vi "capex if then.vi"() -> ()   [LabVIEW 2013]
panel:
  out "Subsystem to set":u16=5
  out "Condition true":bool=TRUE
  out "number outputs":dbl[](array[numeric])
  out "boolean outputs":bool[](array[boolean])=[TRUE, FALSE, FALSE, FALSE]
  out "evaluation value":dbl=1.0
  out "Single value":dbl=23.041248306433495
  in  "stop":bool
  out "SHared variables":dbl[](array[numeric])=[-55770.42973935589, -55770.42973935589, -55770.42973935589, -55770.42973935589, -55753.68398615968, -55753.68398615968, -55753.68398615968, 23.041248306433495]
  in  "Number of criteria":dbl=1.0
  in  "Cluster":T1={"subsystem to check"=7, "Module"=5, "Channel"=7, "criteria"=2, "evaluation value"=1.0, "Subsystem to set"=5, "Set value"=1.0, "Set channel"=0, "Set module"=1} {"Set module" items=["Mod1"=1, "Mod2"=2, "Mod3"=3, "Mod4"=4, "Mod5"=5]; "Set channel" items=["1", "2", "3", "4", "5", "6", "7", "8", "9", "10", "11", "12", "13", "14", "15", "16", "17", "18", "19", "20", "21", "22", "23", "24", "25", "26", "27", "28", "29", "30", "31", "32"]; "Subsystem to set" items=["GPIO"=0, "Chamber temperature"=1, "Chiller"=2, "Analog out"=3, "DC volts"=5, "AC volts"=6, "Relays"=8]; "criteria" items=["==", "!=", ">", "<", ">=", "<="]; "Channel" items=["1", "2", "3", "4", "5", "6", "7", "8", "9", "10", "11", "12", "13", "14", "15", "16", "17", "18", "19", "20", "21", "22", "23", "24", "25", "26", "27", "28", "29", "30", "31", "32"]; "Module" items=["Mod1"=1, "Mod2"=2, "Mod3"=3, "Mod4"=4, "Mod5"=5]; "subsystem to check" items=["GPIO"=0, "chamber temp"=1, "chiller PV"=2, "analog in"=4, "thermocouples"=7, "disabled"=9]}
  # "error: rings need to have full complement of devices but I want to hide some"
  # "GPIO needs more work to be implemented\nSet to \"disabled\" to temporarily disable the criteria from being checked\nIf only one device, leave module set to 1"
  # "Use 0 for off\nand 1 for on\nfor relays"
  # "Little chamber = module 1\nBig chamber = module 2"
  # "gets set to"
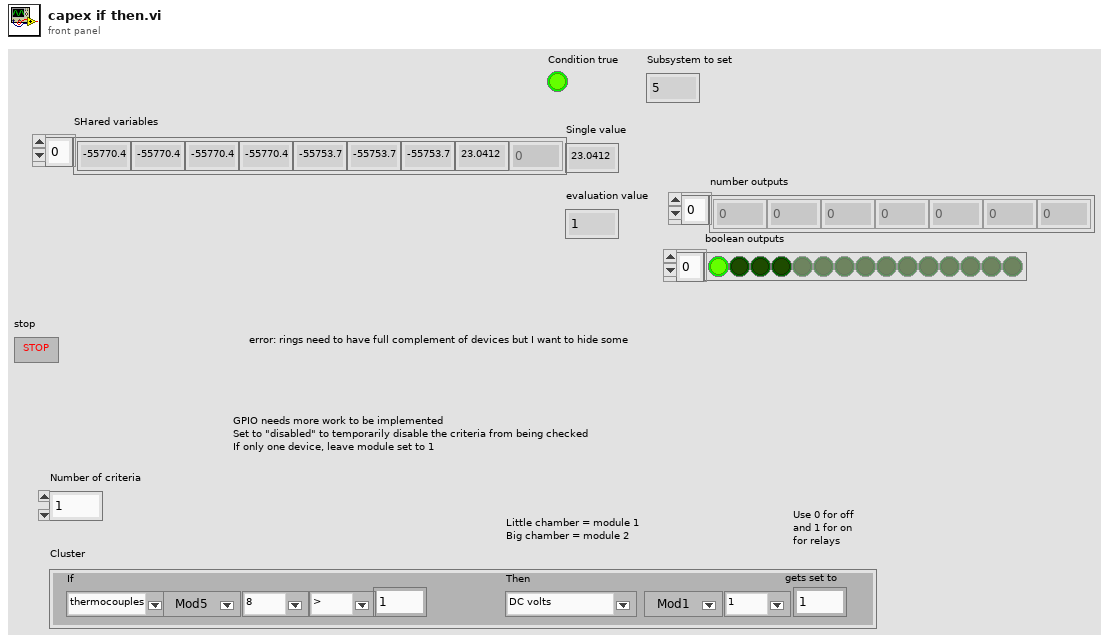
[diagram p1: front panel]
types:
  T1 = cluster{"subsystem to check":u16, "Module":u16, "Channel":u16, "criteria":u16, "evaluation value":dbl, "Subsystem to set":u16, "Set value":dbl, "Set channel":u16, "Set module":u16}
  T2 = cluster{"subsystem to check":u16, "Module":u16, "Channel":u16, "criteria":u16, "evaluation value":dbl, "Subsystem to set":u16, "Set value":dbl, "Set channel":u16, "Set module":u16}[]
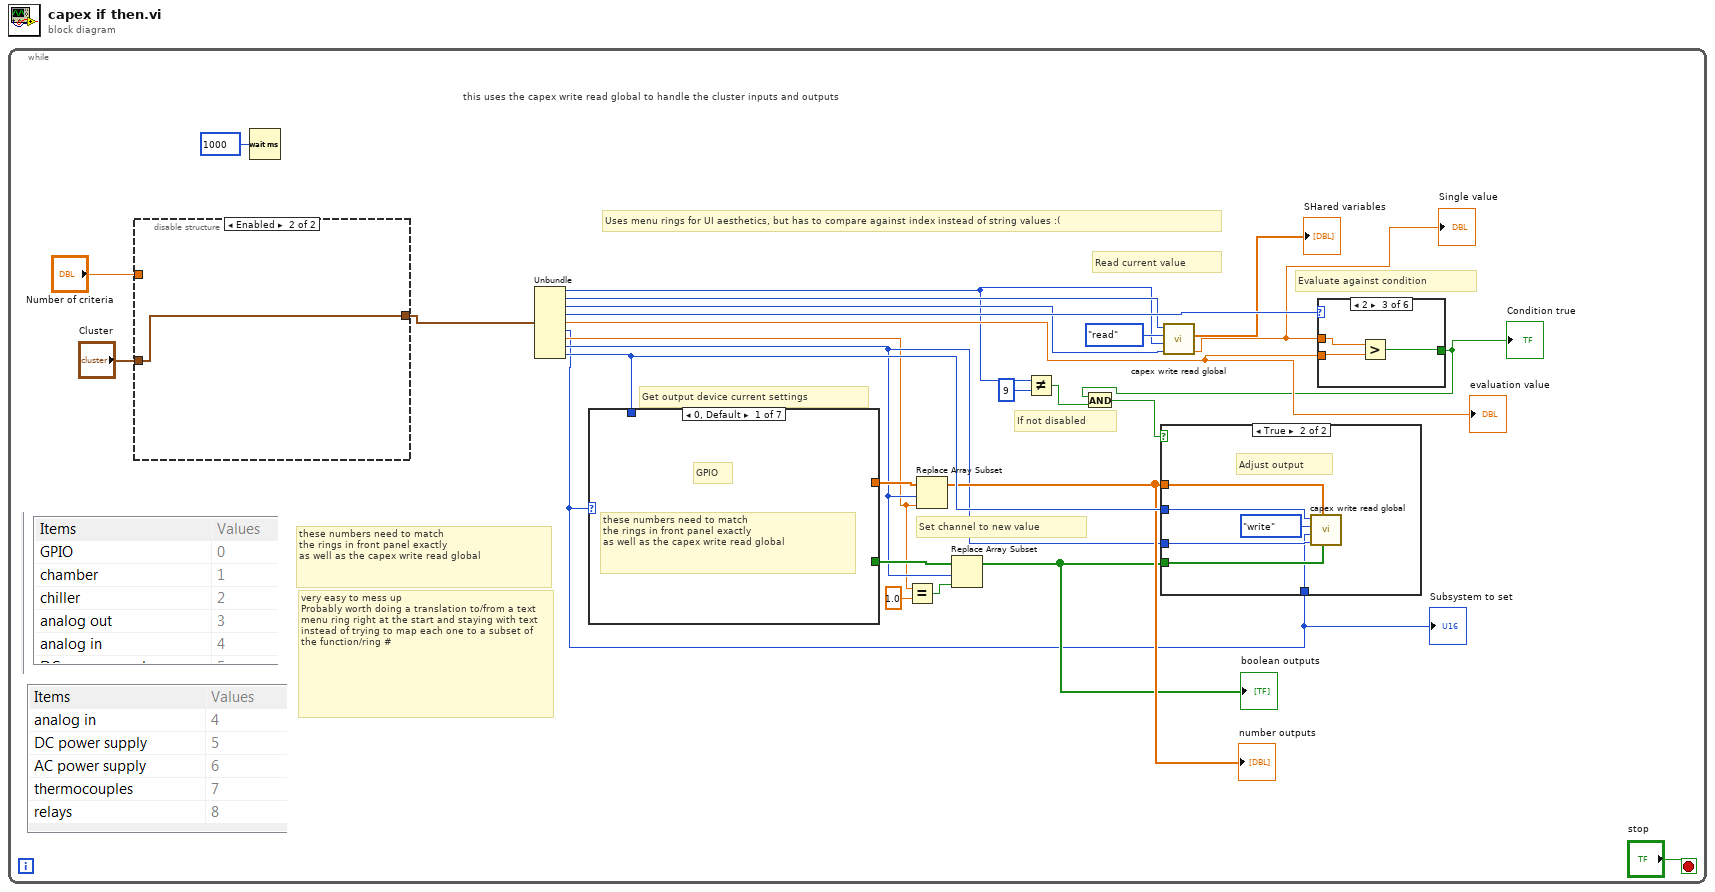
[diagram p0: block diagram]
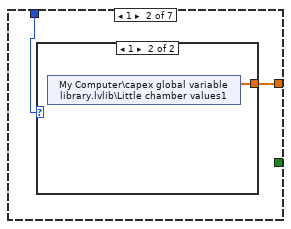
[diagram p2: hidden frame]
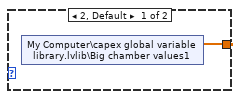
[diagram p3: hidden frame]
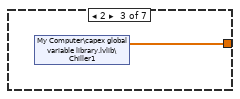
[diagram p4: hidden frame]
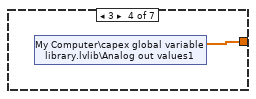
[diagram p5: hidden frame]
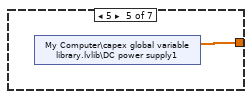
[diagram p6: hidden frame]
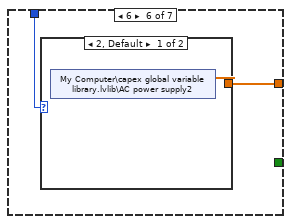
[diagram p7: hidden frame]
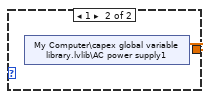
[diagram p8: hidden frame]
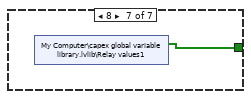
[diagram p9: hidden frame]
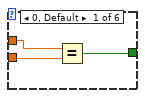
[diagram p11: hidden frame]
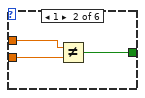
[diagram p12: hidden frame]
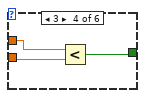
[diagram p13: hidden frame]
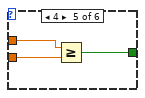
[diagram p14: hidden frame]
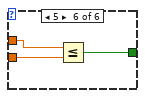
[diagram p15: hidden frame]
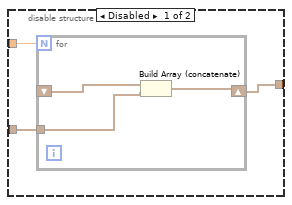
[diagram p16: hidden frame]
diagram:
  n1 = while {
    stop <- "stop" stop-if-true
    # "very easy to mess up\nProbably worth doing a translation to/from a text menu ring right at the start and staying with text instead of trying to map each one to a subset of the function/ring #"
    # "these numbers need to match\nthe rings in front panel exactly\nas well as the capex write read global"
    # "Uses menu rings for UI aesthetics, but has to compare against index instead of string values :("
    # "If not disabled"
    # "Set channel to new value"
    # "Evaluate against condition"
    # "Read current value"
    # "Get output device current settings"
    # "this uses the capex write read global to handle the cluster inputs and outputs"
    n2 = disable-structure shown="Enabled" {
      disable-tunnel: "Number of criteria" -> [w66 _]
      disable-tunnel: "Cluster" -> [w65 w70]
      disable-tunnel: [w64 w70] -> w25
      frame Disabled {
        n3 = for {
          N: w66 -> [_]
          shift-right: [w67] -> w64
          shift-left: _ -> [w68]
          tunnel: w65 -> [w69]
          n4 = Build Array (concatenate)(w68, w69) -> (w67:T2)
        }
      }
      frame Enabled {
      }
    }
    n5 = Wait (ms)(milliseconds to wait=u32 1000) -> ()  [unwired: 1 out]
    n6 = Unbundle(w25) -> ("subsystem to check"=w7:u16, "Module"=w19:u16, "Channel"=w20:u16, "criteria"=w22:u16, "evaluation value"=w18:dbl, "Subsystem to set"=w8:u16, "Set value"=w11:dbl, "Set channel"=w13:u16, "Set module"=w17:u16)
    "evaluation value" <- w18
    "Subsystem to set" <- w8
    n7 = case shown="0, Default" w8 {
      tunnel: w17 -> [_ w29 _ _ _ w36 _]
      tunnel: [_ w28 w32 w33 w34 w35 _] -> w16
      tunnel: [_ _ _ _ _ _ w39] -> w14
      frame 0, Default {
        # "these numbers need to match\nthe rings in front panel exactly\nas well as the capex write read global"
        # "GPIO"
      }
      frame 1 {
        n8 = case shown="1" w29 {
          tunnel: [w30 w31] -> w28
          frame 2, Default {
            n9 = shared-variable "My Computer\\capex global variable library.lvlib\\Big chamber values1"() -> (w30:dbl[])  [unwired: 1 in, 1 out]
          }
          frame 1 {
            n10 = shared-variable "My Computer\\capex global variable library.lvlib\\Little chamber values1"() -> (w31:dbl[])  [unwired: 1 in, 1 out]
          }
        }
      }
      frame 2 {
        n11 = shared-variable "My Computer\\capex global variable library.lvlib\\Chiller1"() -> (w32:dbl[])  [unwired: 1 in, 1 out]
      }
      frame 3 {
        n12 = shared-variable "My Computer\\capex global variable library.lvlib\\Analog out values1"() -> (w33:dbl[])  [unwired: 1 in, 1 out]
      }
      frame 5 {
        n13 = shared-variable "My Computer\\capex global variable library.lvlib\\DC power supply1"() -> (w34:dbl[])  [unwired: 1 in, 1 out]
      }
      frame 6 {
        n14 = case shown="2, Default" w36 {
          tunnel: [w37 w38] -> w35
          frame 2, Default {
            n15 = shared-variable "My Computer\\capex global variable library.lvlib\\AC power supply2"() -> (w37:dbl[])  [unwired: 1 in, 1 out]
          }
          frame 1 {
            n16 = shared-variable "My Computer\\capex global variable library.lvlib\\AC power supply1"() -> (w38:dbl[])  [unwired: 1 in, 1 out]
          }
        }
      }
      frame 8 {
        n17 = shared-variable "My Computer\\capex global variable library.lvlib\\Relay values1"() -> (w39:bool[])  [unwired: 1 in, 1 out]
      }
    }
    n18 = Equal?(x=w11, y=1.0) -> (x = y?=w10:bool)
    n19 = Replace Array Subset(array=w16, new element=w11, index=w13) -> (w15:dbl[])
    "number outputs" <- w15
    n20 = Replace Array Subset(array=w14, new element=w10, index=w13) -> (w9:bool[])
    "boolean outputs" <- w9
    n21 = Not Equal?(x=w7, y=u16 9) -> (x != y?=w5:bool)
    n22 = call "capex write read global.vi"("Channel"=w20, "Subsystem"=w7, "read/write"=enum16{"read", "write"}."read", "Module"=w19) -> ("Single value"=w1:dbl, "Value out"=→"SHared variables":dbl[])  [unwired: 4 in, 2 out]
    "Single value" <- w1
    n23 = case shown="2" w22 {
      tunnel: w1 -> [w48 w51 w54 w57 w60 w63]
      tunnel: w18 -> [w47 w50 w53 w56 w59 w62]
      tunnel: [w46 w49 w52 w55 w58 w61] -> w3
      frame 0, Default {
        n24 = Equal?(x=w48, y=w47) -> (x = y?=w46:bool)
      }
      frame 1 {
        n25 = Not Equal?(x=w51, y=w50) -> (x != y?=w49:bool)
      }
      frame 2 {
        n26 = Greater?(x=w54, y=w53) -> (0:w52:bool)
      }
      frame 3 {
        n27 = Less?(x=w57, y=w56) -> (x < y?=w55:bool)
      }
      frame 4 {
        n28 = Greater Or Equal?(x=w60, y=w59) -> (x >= y?=w58:bool)
      }
      frame 5 {
        n29 = Less Or Equal?(x=w63, y=w62) -> (x <= y?=w61:bool)
      }
    }
    "Condition true" <- w3
    n30 = And(x=w3, y=w5) -> (x .and. y?=w4:bool)
    n31 = case shown="True" w4 {
      tunnel: w17 -> [_ w44]
      tunnel: w13 -> [_ w43]
      tunnel: w15 -> [_ w42]
      tunnel: w9 -> [_ w41]
      tunnel: w8 -> [_ w40]
      frame False {
      }
      frame True {
        # "Adjust output"
        n32 = call "capex write read global.vi"("Bool in"=w41, "Value in"=w42, "Channel"=w43, "Subsystem"=w40, "read/write"=enum16{"read", "write"}."write", "Module"=w44) -> ()  [unwired: 2 in, 4 out]
      }
    }
  }
